vi "Debug Pop Up.vi"(6 "Input":refnum<class>, 9 "Method":string, 10 "Alias":string) -> (4 "Output":refnum<class>)   [LabVIEW 2021, in "jettl.lvlib"]
uses:
  jettl.lvlib
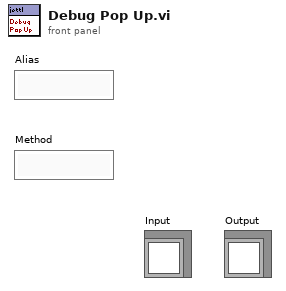
[diagram p1: front panel]
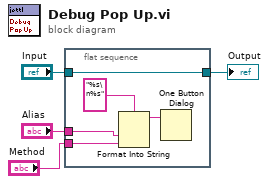
[diagram p0: block diagram]
diagram:
  n1 = flat-sequence {
    tunnel: [w9] -> w1
    tunnel: "Input" -> [w9]
    tunnel: "Method" -> [w5]
    tunnel: "Alias" -> [w6]
    frame #0 {
      n2 = Format Into String(format string="%s\n%s", w6, w5) -> (resulting string=w7:string)  [unwired: 2 in, 1 out]
      n3 = One Button Dialog(message=w7) -> ()  [unwired: 1 in, 1 out]
    }
  }
  "Output" <- w1
